vi "Load Pictures.vi"() -> ()   [LabVIEW 2020, in "VolatusGUIControls.lvlib"]
uses:
  VolatusGUIControls.lvlib
panel:
  in  "Clear":bool
  out "Picture":picture
  in  "path to PNG file":path
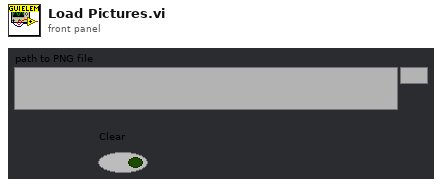
[diagram p1: front panel]
types:
  T1 = typedef "imagedata.ctl" = cluster{"image type":i32, "image depth":i32, "image":u8[], "mask":u8[], "colors":u32[], "Rectangle":cluster{"left":i16, "top":i16, "right":i16, "bottom":i16}}
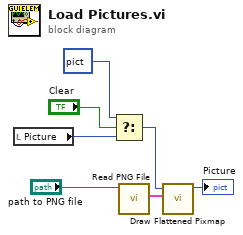
[diagram p0: block diagram]
diagram:
  n1 = local read "Picture"() -> (w4:picture)
  n2 = Select(t=picture data[5B] ("picture"), s="Clear", f=w4) -> (s? t:f=w1:picture)
  n3 = call <vilib>:"Read PNG File.vi"("path to PNG file"="path to PNG file") -> ("image data"=w6:T1)  [unwired: 8 in, 2 out]
  n4 = call <vilib>:"Draw Flattened Pixmap.vi"("image data"=w6, "picture"=w1) -> ("new picture"=→"Picture":picture)  [unwired: 7 in]
